vi "Check Other Machines for Schedule Time.vi"(9 "Processing Time of the Job on This Machine":u16, 10 "Current Machine Available Time":i32, 11 "Time Interval List":T1[](array[typedef])) -> (3 "Time to schedule":i32)   [LabVIEW 2013, in "GanntChart.lvclass"]
uses:
  GanntChart.lvclass
  Controls/Time_Interval_List_Element.ctl
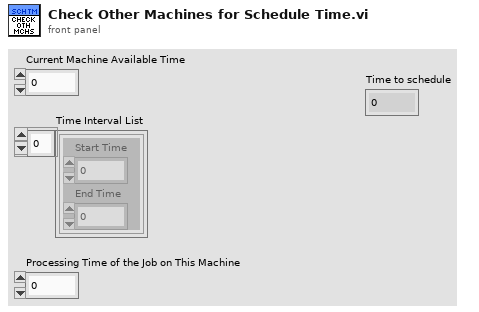
[diagram p1: front panel]
types:
  T1 = typedef "Time_Interval_List_Element.ctl" = cluster{"Start Time":i32, "End Time":i32}
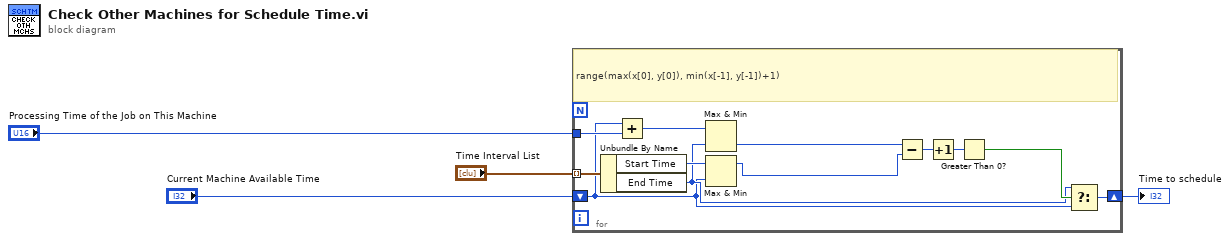
[diagram p0: block diagram]
diagram:
  n1 = for {
    tunnel: "Time Interval List" -> [w16] mode=indexing
    shift-right: [w6] -> w1
    shift-left: "Current Machine Available Time" -> [w5]
    tunnel: "Processing Time of the Job on This Machine" -> [w15]
    # "range(max(x[0], y[0]), min(x[-1], y[-1])+1)"
    n2 = Unbundle By Name(w16) -> ("Start Time"=w14:i32, "End Time"=w7:i32)
    n3 = Add(x=w5, y=w15) -> (x+y=w13:i32)
    n4 = Max & Min(x=w13, y=w7) -> (min(x,y)=w12:i32)  [unwired: 1 out]
    n5 = Max & Min(x=w14, y=w5) -> (max(x,y)=w11:i32)  [unwired: 1 out]
    n6 = Subtract(x=w12, y=w11) -> (x-y=w10:i32)
    n7 = Increment(x=w10) -> (x+1=w9:i32)
    n8 = Greater Than 0?(x=w9) -> (x > 0?=w8:bool)
    n9 = Select(t=w7, s=w8, f=w5) -> (s? t:f=w6:i32)
  }
  "Time to schedule" <- w1
